vi "Set Simulation Mode.vi"(8 "error in (no error)":errorcluster, 11 "Simulate On":bool) -> (0 "error out":errorcluster)   [LabVIEW 2015, in "Tool Interface.lvlib"]
uses:
  Tool Interface.lvlib
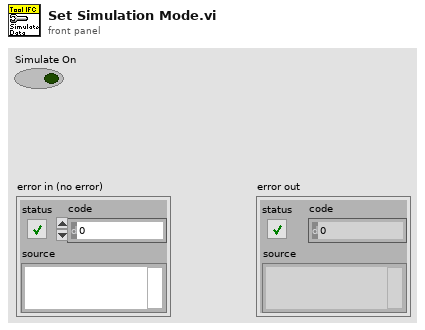
[diagram p1: front panel]
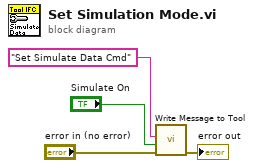
[diagram p0: block diagram]
diagram:
  n1 = call "Write Message to Tool.vi"("error in (no error)"="error in (no error)", "Message Data"="Simulate On", "Message"="Set Simulate Data Cmd") -> ("error out"=→"error out":errorcluster)  [unwired: 8 in]
